vi "AM_PID_tester_basic_data.vi"() -> ()   [LabVIEW 2013]
uses:
  DataMode.ctl
  Input_5782/5782_states.ctl
  <vilib>/Platform/TimedLoop/XDataNode/timing_clust.ctl
  <vilib>/Platform/TimedLoop/XDataNode/nitl_modes.ctl
  <vilib>/Platform/TimedLoop/XDataNode/wakeup.ctl
  <vilib>/rvi/FXPMathLib/FxpConvert/subVIs/nifxpmath_Convert_SimConfig.ctl
  <vilib>/fxp/LVFixedPointQuantizationPolicyTypeDef.ctl
  <vilib>/fxp/LVFixedPointOverflowPolicyTypeDef.ctl
  <vilib>/rvi/Emulation/niFpgaSctlEmulationGetInTimedLoop.vi
  <vilib>/rvi/Emulation/niFpgaEmulationReportErrorSimple.vi
  <vilib>/rvi/Emulation/niFpgaGetClockAttributes.vi
  <vilib>/rvi/eio/common/nirviEmuTemplateMethod_errors.vi
  <vilib>/rvi/Emulation/niFpgaCriticalErrorInLSC.vi
  <vilib>/rvi/DataTransferAndStorage/Register/Emulation/niFpgaRegisterEmulationFpgaImpl.vi
  <instcachedir>/0/niFpgaRegisterEmulationFpgaImpl_DCF4BC0110594B98B44A971D60CEEC4D.lvgen/niFpgaRegisterEmulationFpgaImpl_DCF4BC0110594B98B44A971D60CEEC4D_005.vi
  <vilib>/rvi/DataTransferAndStorage/Container/Common/niFpgaContainerGetUniqueNameForEmu.vi
  <instcachedir>/0/niFpgaRegisterEmulationFpgaImpl_DCF4BC0110594B98B44A971D60CEEC4D.lvgen/niFpgaRegisterEmulationFpgaImpl_DCF4BC0110594B98B44A971D60CEEC4D_016.vi
  <instcachedir>/0/niFpgaRegisterEmulationFpgaImpl_DCF4BC0110594B98B44A971D60CEEC4D.lvgen/niFpgaRegisterEmulationFpgaImpl_DCF4BC0110594B98B44A971D60CEEC4D_017.vi
  <instcachedir>/0/niFpgaRegisterEmulationFpgaImpl_DCF4BC0110594B98B44A971D60CEEC4D.lvgen/niFpgaRegisterEmulationFpgaImpl_DCF4BC0110594B98B44A971D60CEEC4D_012.vi
  <instcachedir>/0/niFpgaRegisterEmulationFpgaImpl_DCF4BC0110594B98B44A971D60CEEC4D.lvgen/niFpgaRegisterEmulationFpgaImpl_DCF4BC0110594B98B44A971D60CEEC4D_015.vi
  <vilib>/rvi/FIFO/Fifo_Resource/nirvififoEmulationReadFpgaImpl.vi
  <vilib>/rvi/interface/RandomDataEmulation/nirviRandomDataMultiElementFPGAFIFO.vi
  <instcachedir>/0/nirviRandomDataMultiElementFPGAFIFO_F2B80EDE0D7944A08478D8D26097D4DB.lvgen/nirviRandomDataMultiElementFPGAFIFO_F2B80EDE0D7944A08478D8D26097D4DB_005.vi
  <vilib>/rvi/interface/RandomDataEmulation/niFpgaRandomDataHandleErrors.vi
  <instcachedir>/0/niFpgaRegisterEmulationFpgaImpl_DCF4BC0110594B98B44A971D60CEEC4D.lvgen/niFpgaRegisterEmulationFpgaImpl_DCF4BC0110594B98B44A971D60CEEC4D_009.vi
  <vilib>/rvi/interface/RandomDataEmulation/nirviRandomDataFPGAFIFO.vi
  <vilib>/rvi/FXPMathLib/FxpConvert/simVIs/DllFxpConvertTemp_sub.vi
  <vilib>/rvi/FIFO/Fifo_Resource/nirvififoEmulationWriteFpgaImpl.vi
  <vilib>/Platform/TimedLoop/XDataNode/XDataNode.xnode
  <vilib>/eio/EIONode/EIONode.xnode
  <vilib>/rvi/DataTransferAndStorage/Container/XNode/niFpgaContainer.xnode
  <vilib>/rvi/DataTransferAndStorage/Register/Emulation/niFpgaRegisterEmulation.vi
  <vilib>/rvi/FIFO/Fifo_Resource/nirvififoEmulationRead.vi
  <vilib>/rvi/interface/RandomDataEmulation/nirviRandomDataFpgaMultiElementTemplate.vi
  <vilib>/rvi/interface/RandomDataEmulation/nirviRandomDataFpgaReadWriteTemplate.vi
  <vilib>/rvi/FXPMathLib/FxpInterpret/XNode/nifxpmath_Interpret.xnode
  <vilib>/rvi/FXPMathLib/FxpConvert/XNode/nifxpmath_Convert.xnode
  <vilib>/rvi/FIFO/Fifo_Resource/nirvififoEmulationWrite.vi
  <vilib>/rvi/FXPMathLib/FxpSub/XNode/nifxpmath_Sub.xnode
  <vilib>/Platform/TimedLoop/XDataNode/XDNodeRunTimeDep.lvlib
  <vilib>/rvi/FXPMathLib/sim/FxpSim.dll
panel:
  in  "AM phase":fxp<+,64,64>
  in  "Continuous":bool
  in  "Downsample":fxp<+,8,8>=1.0
  in  "new coeffs":bool
  in  "FIR coeffs":fxp<+/-,18,18>[](array[numeric])
  in  "CIC Gain":fxp<+/-,32,1>=0.00390625 format="%#_32g"
  in  "Acquisition running":bool
  in  "Phase output":fxp<+,64,64>[](array[numeric])=[0.0, 0.0, 0.0, 0.0, 0.0, 0.0, 0.0, 0.0]
  in  "Simulated phase 5782":fxp<+,64,64>[](array[numeric])=[0.0, 0.0]
  in  "Mode":T1
  in  "Phase 5782":fxp<+,64,64>[](array[numeric])=[0.0, 0.0]
  out "IO Module\\Trigger Input":bool
  in  "IO Module\\AO Data Sync":bool=TRUE
  in  "IO Module\\SPI Write Data":u16
  out "IO Module\\SPI Read Data":u8
  in  "IO Module\\SPI Read":bool
  in  "IO Module\\SPI Write":bool
  in  "IO Module\\SPI Address":u16
  in  "IO Module\\SPI Device":u8
  out "IO Module\\SPI Idle":bool
  in  "delay phase":fxp<+,64,64>
  in  "User Command Commit":bool
  in  "User Command":u8
  out "User Command Idle":bool
  out "User Command Status":u8
  in  "User Data 0":u8
  in  "User Data 1":u8
  out "PLL Locked":bool
  out "User Error":bool
  out "Configured?":bool
  in  "5782 record length":u16=4000 caption="Samples Per Trigger" min=1 step=1
  in  "Trigger Acquisition":bool
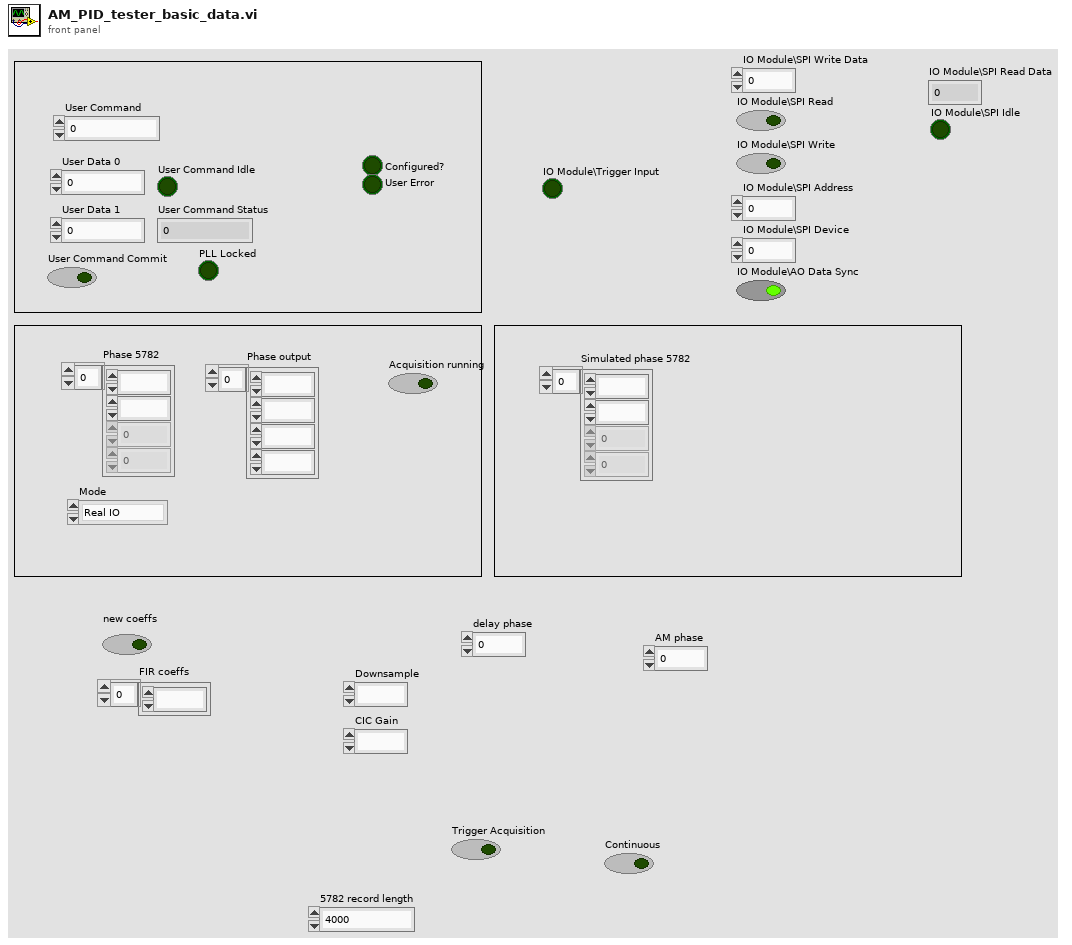
[diagram p1: front panel]
types:
  T1 = typedef "DataMode.ctl" = enum16{"Real IO", "Simulated"}
  T2 = typedef "5782_states.ctl" = enum8{"Wait for trigger", "Acquisition", "Send record length", "Quiet period"}
  T3 = typedef "XDNodeRunTimeDep.lvlib/timing_clust.ctl" = cluster{"Expected End [f-1]":u64, "Actual End [f-1]":u64, "Finished Late? [f-1]":bool, "Expected End [i-1]":u64, "Actual End [i-1]":u64, "Finished Late? [i-1]":bool, "Expected Start [i]":u64, "Actual Start [i]":u64, "Expected Start [f]":u64, "Actual Start [f]":u64, "Source Name":string, "Structure Name":string, "Period":i64, "Deadline":i64, "Offset":i64, "Start":i64, "Priority":i32, "Timeout":i32, "Mode":T4, "Wakeup Reason":T5, "Error":errorcluster, "Source Type":string, "Secondary Source Type":string, "Global End Time":u64, "Global Start Time":u64, "Frame Duration":u64, "Iteration Duration":u64, "Assigned CPU":i32, "I/O Scan Engine Mode":u32}
  T4 = typedef "XDNodeRunTimeDep.lvlib/nitl_modes.ctl" = enum32{"No Change", "Process missed periods, maintain original phase", "Discard missed periods, maintain original phase", "Process missed periods, ignore original phase", "Discard missed periods, ignore original phase"}
  T5 = typedef "XDNodeRunTimeDep.lvlib/wakeup.ctl" = enum32{"Normal", "Aborted", "Asynchronous wakeup", "Timing source error", "Timed loop error", "Timeout"}
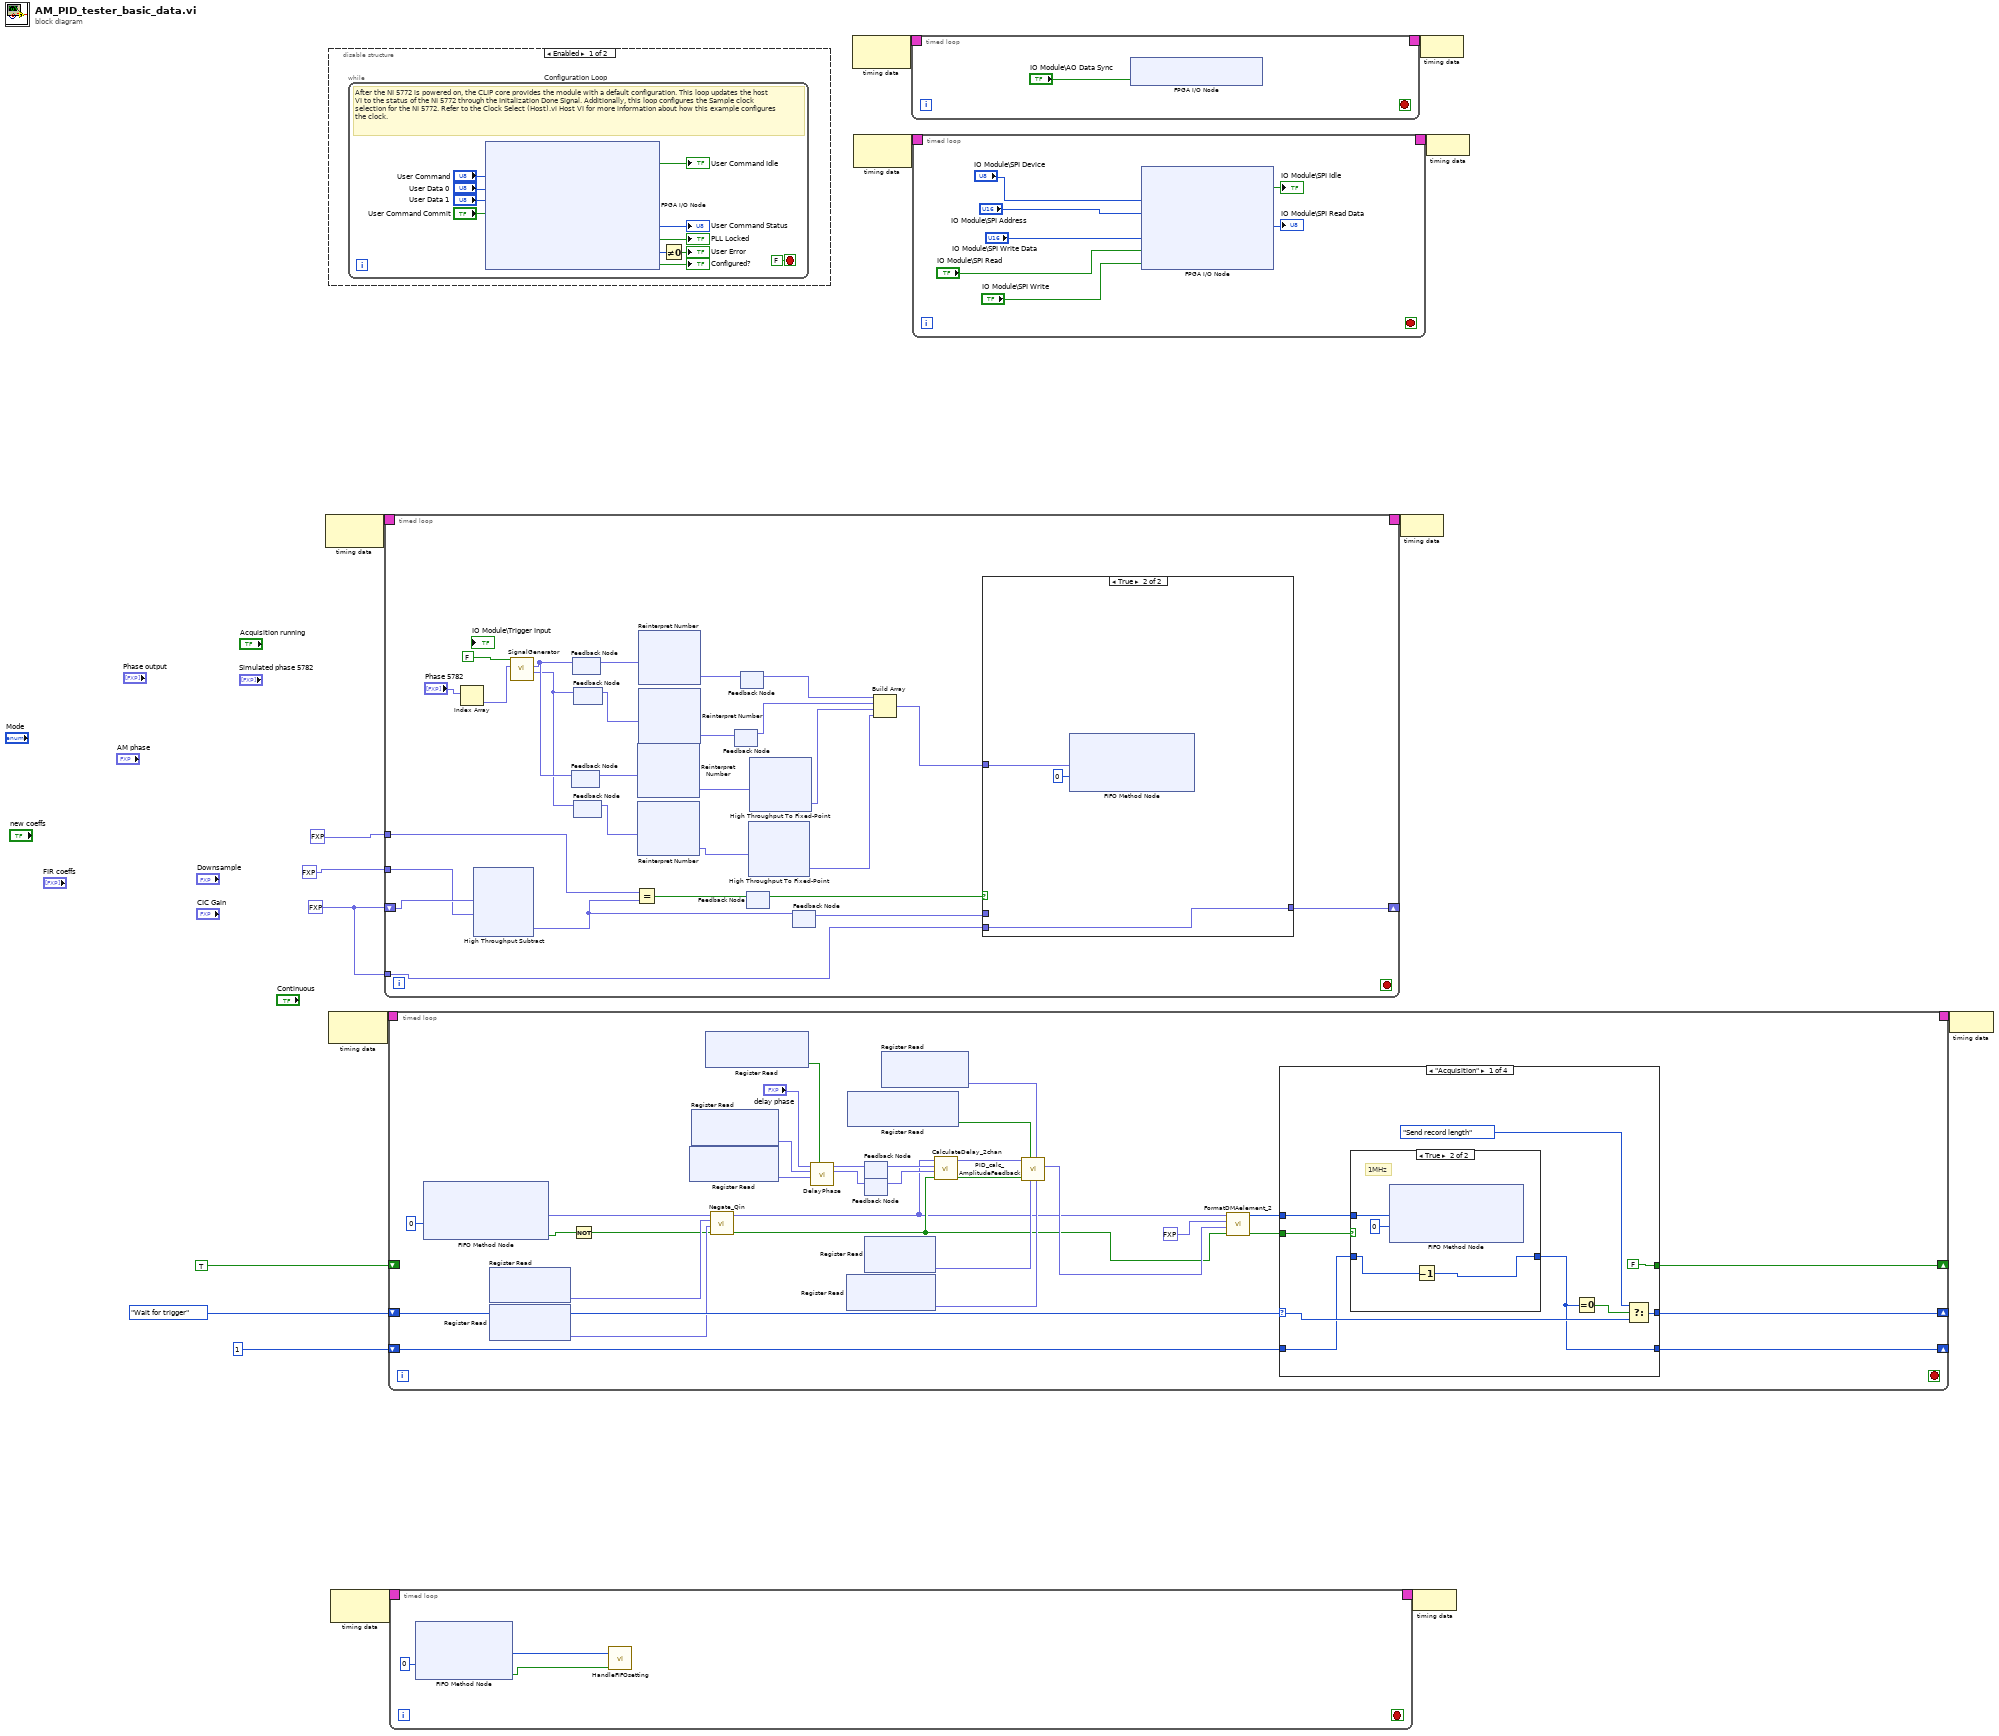
[diagram p0: block diagram]
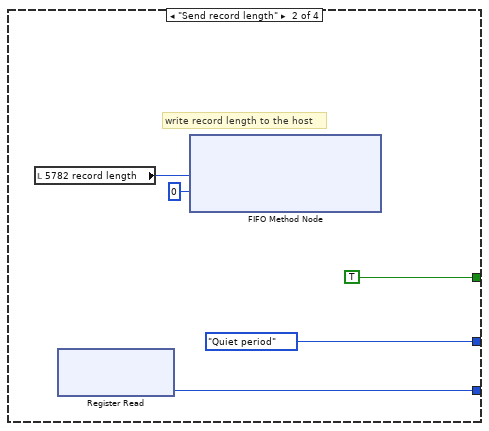
[diagram p4: hidden frame]
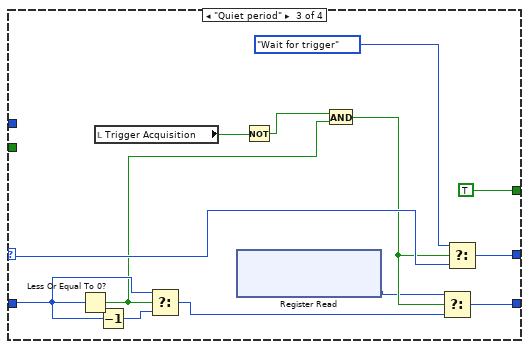
[diagram p5: hidden frame]
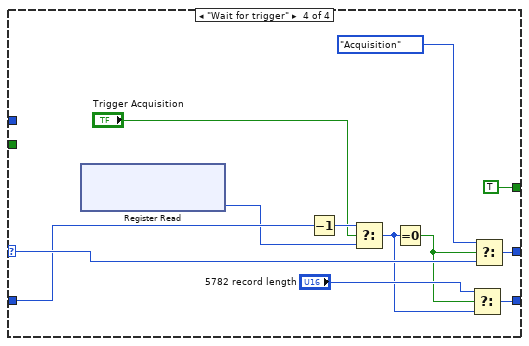
[diagram p6: hidden frame]
diagram:
  w3 = fxp<+/-,8,8> 5.0 ("x")
  n1 = node-c288() -> (w2:T3)  [unwired: 1 in]
  n2 = disable-structure shown="Enabled" {
    frame Enabled {
      n3 = while "Configuration Loop" {
        stop <- FALSE stop-if-true
        # "After the NI 5772 is powered on, the CLIP core provides the module with a default configuration. This loop updates the host VI to the status of the NI 5772 through the Initalization Done Signal. Additionally, this loop configures the Sample clock selection for the NI 5772. Refer to the Clock Select (Host).vi Host VI for more information about how this example configures the clock."
        n4 = xnode "FPGA I/O Node"("IO Module\\User Command"="User Command", "IO Module\\User Data 0"="User Data 0", "IO Module\\User Data 1"="User Data 1", "IO Module\\User Command Commit"="User Command Commit") -> ("IO Module\\User Command Idle"=→"User Command Idle":bool, "IO Module\\User Command Status"=→"User Command Status":u8, "IO Module\\PLL Locked"=→"PLL Locked":bool, "IO Module\\User Error"=w22:u8, "IO Module\\Initialization Done"=→"Configured?":bool)  [unwired: 9 in, 9 out]
        n5 = Not Equal To 0?(x=w22) -> (x != 0?=→"User Error":bool)
      }
    }
    frame Disabled {
    }
  }
  n6 = node-c288() -> (w16:T3)  [unwired: 1 in]
  n7 = node-c288() -> (w11:T3)  [unwired: 1 in]
  n8 = timed-loop {
    shift-right: [w50] -> _
    shift-left: w3 -> [w54]
    tunnel: fxp<+/-,8,8> 1.0 ("y") -> [w53]
    tunnel: fxp<+/-,8,8> 0.0 ("y") -> [w52]
    tunnel: w3 -> [w51]
    timing: w2 -> [_]
    timing-out: [_] -> w1
    stop <- _ stop-if-true
    n9 = Index Array(array="Phase 5782") -> (element=w28:fxp<+,64,64>)  [unwired: 1 in]
    n10 = xnode "High Throughput Subtract"("x"=w54, "y"=w53) -> ("x-y"=w47:fxp<+/-,8,8>)
    n11 = call "SignalGenerator.vi"("phase"=w28, "Reset"=FALSE) -> ("Cos"=w39:fxp<+/-,16,0>, "Sin"=w40:fxp<+/-,16,0>)  [unwired: 7 in, 1 out]
    n12 = feedback #1() -> (w41:fxp<+/-,16,0>)  [unwired: 1 in]
    n13 = feedback-in #1(w40) -> ()
    n14 = feedback #2() -> (w44:fxp<+/-,16,0>)  [unwired: 1 in]
    n15 = feedback-in #2(w40) -> ()
    n16 = feedback #3() -> (w42:fxp<+/-,16,0>)  [unwired: 1 in]
    n17 = feedback-in #3(w39) -> ()
    n18 = feedback #4() -> (w43:fxp<+/-,16,0>)  [unwired: 1 in]
    n19 = feedback-in #4(w39) -> ()
    n20 = Equal?(x=w52, y=w47) -> (x = y?=w49:bool)
    n21 = xnode "Reinterpret Number"("x"=w41) -> ("y"=w38:fxp<+/-,16,15>)
    n22 = xnode "Reinterpret Number"("x"=w42) -> ("y"=w37:fxp<+/-,16,15>)
    n23 = xnode "Reinterpret Number"("x"=w44) -> ("y"=w36:fxp<+/-,16,14>)
    n24 = xnode "Reinterpret Number"("x"=w43) -> ("y"=w35:fxp<+/-,16,14>)
    n25 = feedback #5() -> (w33:fxp<+/-,16,14>)  [unwired: 1 in]
    n26 = feedback-in #5(w35) -> ()
    n27 = feedback #6() -> (w34:fxp<+/-,16,14>)  [unwired: 1 in]
    n28 = feedback-in #6(w36) -> ()
    n29 = feedback #7() -> (w48:bool)  [unwired: 1 in]
    n30 = feedback-in #7(w49) -> ()
    n31 = xnode "High Throughput To Fixed-Point"("x"=w37) -> ("y"=w31:fxp<+/-,16,14>)
    n32 = xnode "High Throughput To Fixed-Point"("x"=w38) -> ("y"=w32:fxp<+/-,16,14>)
    n33 = feedback #8() -> (w46:fxp<+/-,8,8>)  [unwired: 1 in]
    n34 = feedback-in #8(w47) -> ()
    n35 = Build Array(w34, w33, w32, w31) -> (w30:fxp<+/-,16,14>[])
    n36 = case shown="True" w48 {
      tunnel: w51 -> [_ w102]
      tunnel: w46 -> [w99 _]
      tunnel: [w99 w102] -> w50
      tunnel: w30 -> [_ w100]
      frame False {
      }
      frame True {
        n37 = xnode ("FIFO Method Node")("Element"=w100, "Timeout"=0) -> ()  [unwired: 1 in, 2 out]
      }
    }
  }
  n38 = timed-loop {
    timing: w16 -> [_]
    timing-out: [_] -> w15
    shift-right: [w133] -> _
    shift-left: 5782_states."Wait for trigger" ("5782 states") -> [w135]
    shift-right: [w132] -> _
    shift-left: u16 1 ("trigger samples") -> [w134]
    shift-right: [w127] -> _
    shift-left: TRUE -> [_]
    stop <- _ stop-if-true
    n39 = xnode ("FIFO Method Node")("Timeout"=0) -> ("Element"=w109:fxp<+/-,16,14>[], "Timed Out?"=w130:bool)  [unwired: 1 in, 1 out]
    n40 = xnode ("Register Read")() -> ("Data"=w120:fxp<+/-,16,14>)  [unwired: 1 in, 1 out]
    n41 = xnode ("Register Read")() -> ("Data"=w121:fxp<+/-,16,14>)  [unwired: 1 in, 1 out]
    n42 = Not(x=w130) -> (.not. x?=w110:bool)
    n43 = xnode ("Register Read")() -> ("Data"=w117:fxp<+/-,16,0>)  [unwired: 1 in, 1 out]
    n44 = xnode ("Register Read")() -> ("Data"=w118:fxp<+/-,16,0>)  [unwired: 1 in, 1 out]
    n45 = xnode ("Register Read")() -> ("Data"=w119:bool)  [unwired: 1 in, 1 out]
    n46 = call "Negate_Qin.vi"("valid in"=w110, "DC offset chan 1"=w120, "DC offset chan 0"=w121, "Data in"=w109) -> ("valid out"=w106:bool, "Data out"=w105:fxp<+/-,16,14>[])  [unwired: 6 in]
    n47 = call "DelayPhase.vi"("Use fixed delay"=w119, "fixed cos_fi"=w117, "fixed sin fi"=w118, "delay phase"="delay phase") -> ("cos_fi"=w122:fxp<+/-,16,0>, "sin fi"=w123:fxp<+/-,16,0>)  [unwired: 6 in]
    n48 = xnode ("Register Read")() -> ("Data"=w112:fxp<+/-,32,6>)  [unwired: 1 in, 1 out]
    n49 = xnode ("Register Read")() -> ("Data"=w114:bool)  [unwired: 1 in, 1 out]
    n50 = feedback-in #9(w123) -> ()
    n51 = feedback #9() -> (w126:fxp<+/-,16,0>)  [unwired: 1 in]
    n52 = feedback #10() -> (w125:fxp<+/-,16,0>)  [unwired: 1 in]
    n53 = feedback-in #10(w122) -> ()
    n54 = xnode ("Register Read")() -> ("Data"=w113:fxp<+/-,32,6>)  [unwired: 1 in, 1 out]
    n55 = xnode ("Register Read")() -> ("Data"=w111:fxp<+/-,32,6>)  [unwired: 1 in, 1 out]
    n56 = call "CalculateDelay_2chan.vi"("input valid"=w106, "cos_fi"=w125, "sin fi"=w126, "Data in"=w105) -> ("output valid"=w115:bool, "Data out"=w116:fxp<+/-,16,14>[])  [unwired: 6 in]
    n57 = call "PID_calc_AmplitudeFeedback.vi"("Kd/Tau"=w112, "Ki*Tau"=w111, "Kp"=w113, "Enabled"=w114, "input valid"=w115, "Data in"=w116) -> ("c(t)"=w108:fxp<+/-,32,21>)  [unwired: 2 in, 3 out]
    n58 = call "FormatDMAelement_2.vi"("valid in"=w106, "c(t) - AM"=w108, "c(t) - Phase"=fxp<+/-,32,4> 0.0, "Data in"=w105) -> ("valid out"=w128:bool, "Element"=w129:u64[])  [unwired: 6 in]
    n59 = case shown="\"Acquisition\"" w135 {
      selector: w135 -> [w144 _ w166 w179]
      tunnel: w134 -> [w140 _ w159 w170]
      tunnel: [w143 5782_states."Quiet period" ("5782 states") w165 w178] -> w133
      tunnel: [w137 w150 w167 w177] -> w132
      tunnel: w129 -> [w138 _ _ _]
      tunnel: w128 -> [w139 _ _ _]
      tunnel: [FALSE TRUE TRUE TRUE] -> w127
      frame "Acquisition" {
        n60 = case shown="True" w139 {
          tunnel: w138 -> [_ w149]
          tunnel: [w145 w146] -> w137
          tunnel: w140 -> [w145 w147]
          frame False {
          }
          frame True {
            # "1MHz"
            n61 = xnode ("FIFO Method Node")("Element"=w149, "Timeout"=0) -> ()  [unwired: 1 in, 2 out]
            n62 = Decrement(x=w147) -> (x-1=w146:u16)
          }
        }
        n63 = Equal To 0?(x=w137) -> (x = 0?=w141:bool)
        n64 = Select(t=5782_states."Send record length" ("5782 states"), s=w141, f=w144) -> (s? t:f=w143:T2)
      }
      frame "Send record length" {
        # "write record length to the host"
        n65 = local read "5782 record length"() -> (w151:u16)
        n66 = xnode ("Register Read")() -> ("Data"=w150:u16)  [unwired: 1 in, 1 out]
        n67 = xnode ("FIFO Method Node")("Element"=w151, "Timeout"=0) -> ()  [unwired: 1 in, 2 out]
      }
      frame "Quiet period" {
        n68 = Less Or Equal To 0?(x=w159) -> (x <= 0?=w158:bool)
        n69 = local read "Trigger Acquisition"() -> (w162:bool)
        n70 = Decrement(x=w159) -> (x-1=w160:u16)
        n71 = Select(t=w159, s=w158, f=w160) -> (s? t:f=w157:u16)
        n72 = xnode ("Register Read")() -> ("Data"=w156:u16)  [unwired: 1 in, 1 out]
        n73 = Not(x=w162) -> (.not. x?=w155:bool)
        n74 = And(x=w155, y=w158) -> (x .and. y?=w164:bool)
        n75 = Select(t=w156, s=w164, f=w157) -> (s? t:f=w167:u16)
        n76 = Select(t=5782_states."Wait for trigger" ("5782 states"), s=w164, f=w166) -> (s? t:f=w165:T2)
      }
      frame "Wait for trigger" {
        n77 = xnode ("Register Read")() -> ("Data"=w169:u16)  [unwired: 1 in, 1 out]
        n78 = Decrement(x=w170) -> (x-1=w171:u16)
        n79 = Select(t=w171, s="Trigger Acquisition", f=w169) -> (s? t:f=w172:u16)
        n80 = Equal To 0?(x=w172) -> (x = 0?=w173:bool)
        n81 = Select(t="5782 record length", s=w173, f=w172) -> (s? t:f=w177:u16)
        n82 = Select(t=5782_states."Acquisition" ("5782 states"), s=w173, f=w179) -> (s? t:f=w178:T2)
      }
    }
  }
  n83 = timed-loop {
    timing: w11 -> [_]
    timing-out: [_] -> w10
    stop <- _ stop-if-true
    n84 = xnode ("FIFO Method Node")("Timeout"=0) -> ("Element"=w183:u64, "Timed Out?"=w182:bool)  [unwired: 1 in, 1 out]
    n85 = call "HandleFIFOsetting.vi"("timed out"=w182, "Value"=w183) -> ()  [unwired: 10 in]
  }
  n86 = node-c288() -> (w7:T3)  [unwired: 1 in]
  n87 = node-c288() -> (w9:T3)  [unwired: 1 in]
  n88 = timed-loop {
    timing: w7 -> [_]
    timing-out: [_] -> w6
    stop <- _ stop-if-true
    n89 = xnode "FPGA I/O Node"("IO Module\\AO Data Sync"="IO Module\\AO Data Sync") -> ()  [unwired: 1 in, 1 out]
  }
  n90 = timed-loop {
    timing: w9 -> [_]
    timing-out: [_] -> w8
    stop <- _ stop-if-true
    n91 = xnode "FPGA I/O Node"("IO Module\\SPI Device"="IO Module\\SPI Device", "IO Module\\SPI Address"="IO Module\\SPI Address", "IO Module\\SPI Write Data"="IO Module\\SPI Write Data", "IO Module\\SPI Read"="IO Module\\SPI Read", "IO Module\\SPI Write"="IO Module\\SPI Write") -> ("IO Module\\SPI Idle"=→"IO Module\\SPI Idle":bool, "IO Module\\SPI Read Data"=→"IO Module\\SPI Read Data":u8)  [unwired: 7 in, 7 out]
  }
  n92 = node-c288(w1) -> ()
  n93 = node-c288(w10) -> ()
  n94 = node-c288(w6) -> ()
  n95 = node-c288(w8) -> ()
  n96 = node-c288(w15) -> ()
